vi "CODCr通讯.vi"() -> ()   [LabVIEW 2016, in "CODCr库.lvlib"]
uses:
  <vilib>/Plasmionique/MB Master/MB_Master/MB_Master.lvclass
  <vilib>/Plasmionique/MB Master/MB Master.lvlib
  <vilib>/Utility/config.llb/NI_LVConfig.lvlib
panel:
  out "状态告警区":u16[](array[numeric])
  out "测量数据区":u16[](array[numeric])
  in  "读取参数":bool
  in  "读取数据":bool
  in  "释放串口":bool
  in  "打开串口":bool
  out "队列中元素数量":i32
  out "元素":cluster{"命令":string}[](array[cluster])
  out "待处理插入数量":i32
  out "读取公式":u16[](array[numeric])
  out "读取参数":u16[](array[numeric])
  out "数据存储":u16[](array[numeric])
  out "通讯状态":bool
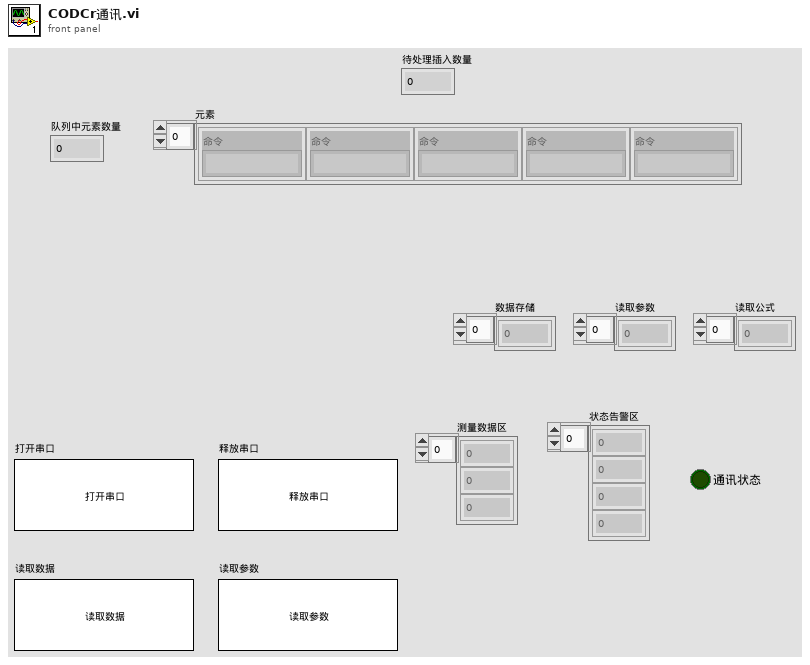
[diagram p1: front panel]
types:
  T1 = typedef "NI_LVConfig.lvlib/Config Data RefNum.ctl" = refnum<k1>
  T2 = cluster{"因子编码":u32, "单位":u16, "标样参考值":sgl, "水样数据时间":timestamp, "水样实测值":sgl, "水样数据标识":string, "标样数据时间":timestamp, "标样实测值":sgl, "标样数据标识":string, "空白数据时间":timestamp, "空白实测值":sgl, "空白数据标识":string, "零点核查数据时间":timestamp, "零点核查实测值":sgl, "零点核查数据标识":string, "跨度核查数据时间":timestamp, "跨度核查实测值":sgl, "跨度核查数据标识":string, "加标回收数据时间":timestamp, "加标回收实测值":sgl, "加标回收数据标识":string, "平行样数据时间":timestamp, "平行样实测值":sgl, "平行样数据标识":string}
  T3 = cluster{"系统时间":timestamp, "工作状态":enum16{"空闲", "水样测试", "标样核查", "零点核查", "跨度核查", "空白测试", "平行样测试", "加标回收", "空白校准", "标样校准", "初始化（清洗）"}, "测量模式":enum16{"待机", "连续模式", "周期模式", "定点模式", "受控模式", "手动模式"}, "告警代码":u16, "故障代码":u16, "日志代码":u16, "软件版本":u16, "F0":sgl, "F1":sgl, "F2":sgl, "F3":sgl, "T":sgl, "H":sgl, "id":u16, "flowid":u16, "量程":u16}
  T4 = cluster{"测量精度":u16, "消解温度":u16, "消解时长":u16, "量程下限":sgl, "量程上限":sgl, "曲线斜率K":sgl, "曲线斜率B":sgl, "标定日期":timestamp, "标液1浓度":sgl, "标液1测量过程值":sgl, "标液2浓度":sgl, "标液2测量过程值":sgl, "标液3浓度":sgl, "标液3测量过程值":sgl, "标液4浓度":sgl, "标液4测量过程值":sgl, "标液5浓度":sgl, "标液5测量过程值":sgl, "线性相关系数":sgl, "试剂余量":u32, "测量滴定值或吸光度":sgl, "空白校准时间":timestamp, "标样校准时间":timestamp, "检出限值":sgl, "校准系数":sgl, "设备系列号":string}
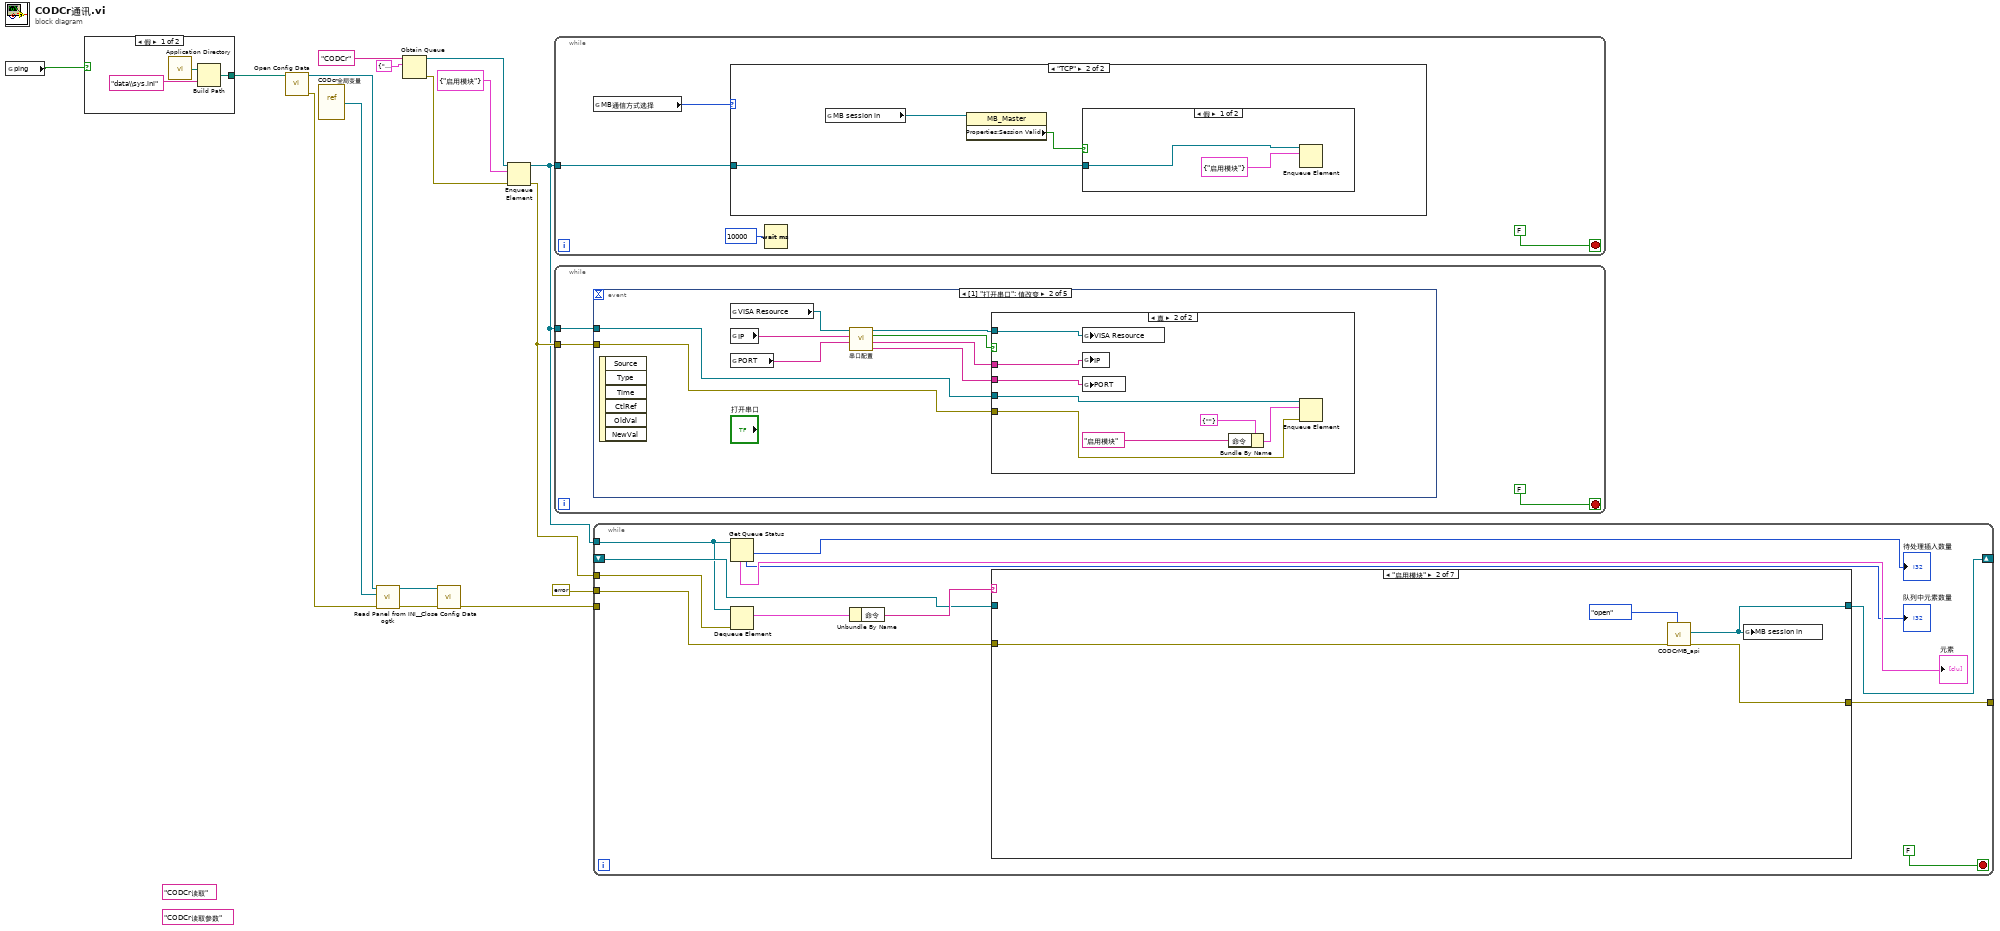
[diagram p0: block diagram]
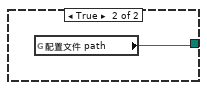
[diagram p2: hidden frame]
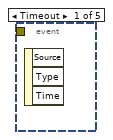
[diagram p5: hidden frame]
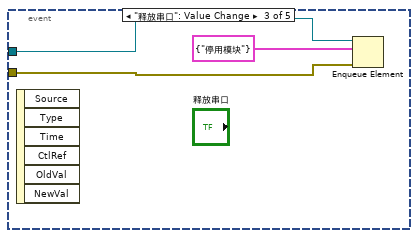
[diagram p7: hidden frame]
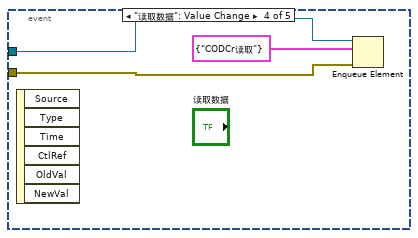
[diagram p8: hidden frame]
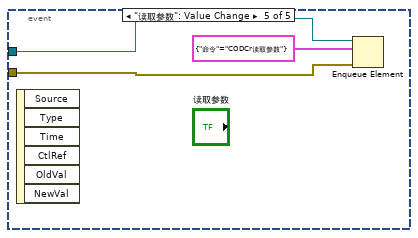
[diagram p9: hidden frame]
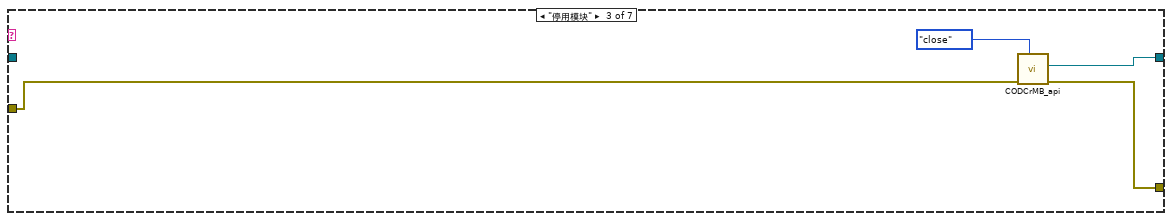
[diagram p11: hidden frame]
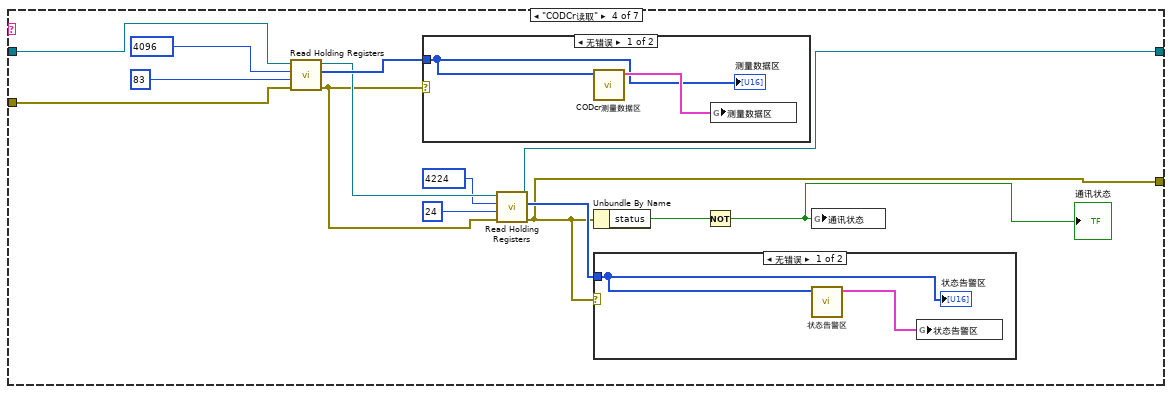
[diagram p12: hidden frame]
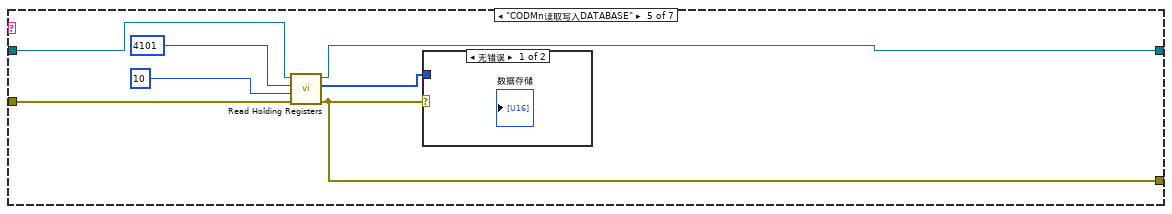
[diagram p15: hidden frame]
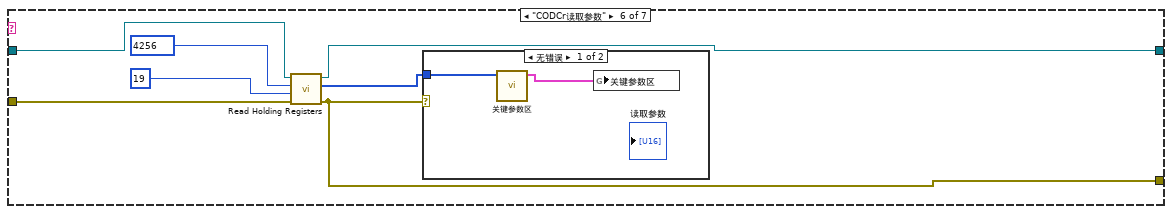
[diagram p17: hidden frame]
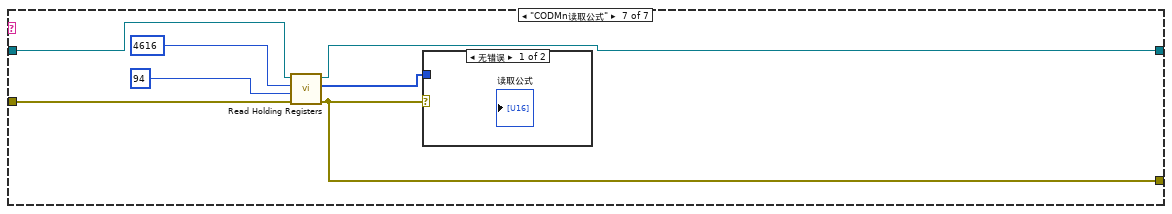
[diagram p19: hidden frame]
diagram:
  (unwired) "CODCr读取参数" ("名称（未命名）")
  (unwired) "CODCr读取" ("名称（未命名）")
  n1 = global read "CODcr全局变量.vi" "ping"() -> (w2:bool)
  n2 = case shown="假" w2 {
    tunnel: [w18 w20] -> w1
    frame False {
      n3 = call <vilib>:"Application Directory.vi"() -> ("Application Directory"=w19:path)
      n4 = Build Path(base path=w19, name or relative path="data\\sys.ini" ("名称或相对路径")) -> (appended path=w18:path)
    }
    frame True {
      n5 = global read "CODcr全局变量.vi" "配置文件 path"() -> (w20:path)
    }
  }
  n6 = call <vilib>:"Open Config Data.vi"("configuration file path"=w1) -> ("error out"=w7:errorcluster, "refnum"=w10:T1)  [unwired: 8 in, 1 out]
  n7 = vi-ref "CODcr全局变量.vi"() -> (w9:refnum<vi>)
  n8 = call <userlib>:"Read Panel from INI__ogtk.vi"("error in (no error)"=w7, "VI ref"=w9, "refnum"=w10) -> ("error out"=w6:errorcluster, "refnum out"=w8:T1)  [unwired: 7 in]
  n9 = Obtain Queue(name (unnamed)="CODCr" ("名称（未命名）"), element data type=cluster{"命令":string} {"命令"="启用模块"} ("元素")) -> (queue out=w13:refnum<queue>, error out=w12:errorcluster)  [unwired: 3 in, 1 out]
  n10 = call <vilib>:"Close Config Data.vi"("error in (no error)"=w6, "refnum"=w8) -> ("error out"=w3:errorcluster)  [unwired: 8 in, 1 out]
  n11 = Enqueue Element(queue=w13, element=cluster{"命令":string} {"命令"="启用模块"} ("元素"), error in (no error)=w12) -> (queue out=w4:refnum<queue>, error out=w5:errorcluster)  [unwired: 1 in, 1 out]
  n12 = while {
    tunnel: w4 -> [w24]
    stop <- FALSE stop-if-true
    n13 = global read "CODcr全局变量.vi" "MB通信方式选择"() -> (w22:enum16{"串口", "TCP"})
    n14 = case shown="\"TCP\"" w22 {
      tunnel: w24 -> [_ w25]
      frame "串口", Default {
      }
      frame "TCP" {
        n15 = global read "CODCr外部API.vi" "MB session in"() -> (w27:refnum<class "MB_Master.lvclass">)
        n16 = property class="MB_Master"(reference=w27) -> ("Properties:Session Valid"=w26:bool)  [unwired: 1 in, 2 out]
        n17 = case shown="假" w26 {
          tunnel: w25 -> [w29 _]
          frame False {
            n18 = Enqueue Element(queue=w29, element=cluster{"命令":string} {"命令"="启用模块"} ("元素")) -> ()  [unwired: 2 in, 3 out]
          }
          frame True {
          }
        }
      }
    }
    n19 = Wait (ms)(milliseconds to wait=u32 10000 ("等待时间（毫秒）")) -> ()  [unwired: 1 out]
  }
  n20 = while {
    tunnel: w4 -> [w31]
    tunnel: w5 -> [w30]
    stop <- FALSE stop-if-true
    n21 = event shown="[1] \"打开串口\": 值改变" {
      selector: _ -> [_ _ _ _ _]
      dyn-events: _ -> [_ _ _ _ _]
      timeout: _ -> [_ _ _ _ _]
      tunnel: w31 -> [_ w41 w52 w54 w57]
      tunnel: w30 -> [_ w40 w51 w53 w56]
      event Timeout {
        n22 = event-data() -> ()  [unwired: 1 in, 3 out]
      }
      event "打开串口": Value Change {
        n23 = event-data() -> ()  [unwired: 1 in, 6 out]
        n24 = global read "CODcr全局变量.vi" "VISA Resource"() -> (w39:refnum<visa-resource-name>)
        n25 = global read "CODcr全局变量.vi" "IP"() -> (w34:string)
        n26 = global read "CODcr全局变量.vi" "PORT"() -> (w33:string)
        n27 = call "串口配置.vi"("PORT"=w33, "IP"=w34, "请选择串口:"=w39) -> ("PORT 2"=w35:string, "IP 2"=w36:string, "确认 2"=w38:bool, "VISA资源名称 2"=w37:refnum<visa-resource-name>)  [unwired: 5 in]
        n28 = case shown="真" w38 {
          tunnel: w37 -> [_ w44]
          tunnel: w41 -> [_ w46]
          tunnel: w40 -> [_ w45]
          tunnel: w36 -> [_ w43]
          tunnel: w35 -> [_ w42]
          frame False {
          }
          frame True {
            n29 = global write "CODcr全局变量.vi" "VISA Resource"(w44) -> ()
            n30 = global write "CODcr全局变量.vi" "IP"(w43) -> ()
            n31 = global write "CODcr全局变量.vi" "PORT"(w42) -> ()
            n32 = Bundle By Name(cluster=cluster{"命令":string} {"命令"=""} ("元素"), "命令"="启用模块" ("名称（未命名）")) -> (w47:cluster{"命令":string})
            n33 = Enqueue Element(queue=w46, element=w47, error in (no error)=w45) -> ()  [unwired: 1 in, 3 out]
          }
        }
      }
      event "释放串口": Value Change {
        n34 = event-data() -> ()  [unwired: 1 in, 6 out]
        n35 = Enqueue Element(queue=w52, element=cluster{"命令":string} {"命令"="停用模块"} ("元素"), error in (no error)=w51) -> ()  [unwired: 1 in, 3 out]
      }
      event "读取数据": Value Change {
        n36 = event-data() -> ()  [unwired: 1 in, 6 out]
        n37 = Enqueue Element(queue=w54, element=cluster{"命令":string} {"命令"="CODCr读取"} ("元素"), error in (no error)=w53) -> ()  [unwired: 1 in, 3 out]
      }
      event "读取参数": Value Change {
        n38 = event-data() -> ()  [unwired: 1 in, 6 out]
        n39 = Enqueue Element(queue=w57, element=cluster{"命令":string} {"命令"="CODCr读取参数"} ("元素"), error in (no error)=w56) -> ()  [unwired: 1 in, 3 out]
      }
    }
  }
  n40 = while {
    tunnel: w4 -> [w62]
    tunnel: w5 -> [w69]
    tunnel: [w63] -> _
    shift-right: [w66] -> _
    shift-left: _ -> [w65]
    tunnel: errorcluster {"status"=FALSE, "code"=0, "source"=""} ("error out") -> [w64]
    tunnel: w3 -> [_]
    stop <- FALSE stop-if-true
    n41 = Get Queue Status(queue=w62) -> (# pending insert=→"待处理插入数量":i32, # elements in queue=→"队列中元素数量":i32, elements=→"元素":cluster{"命令":string}[])  [unwired: 2 in, 5 out]
    n42 = Dequeue Element(queue=w62, error in (no error)=w69) -> (element=w68:cluster{"命令":string})  [unwired: 1 in, 3 out]
    n43 = Unbundle By Name(w68) -> ("命令"=w67:string)
    n44 = case shown="\"启用模块\"" w67 {
      tunnel: [w72 w73 w77 w88 w101 w109 w118] -> w66
      tunnel: [w71 w76 w78 w81 w99 w108 w117] -> w63
      tunnel: w65 -> [w72 _ _ w94 w105 w112 w121]
      tunnel: w64 -> [w71 w74 w79 w93 w102 w111 w120]
      frame Default {
      }
      frame "启用模块" {
        n45 = call "CODCrMB_api.vi"("STEP"=enum16{"open", "read", "write", "close"}."open", "Error in"=w74) -> ("error out"=w76:errorcluster, "MB session out"=w73:refnum<class "MB_Master.lvclass">)  [unwired: 7 in, 1 out]
        n46 = global write "CODCr外部API.vi" "MB session in"(w73) -> ()
      }
      frame "停用模块" {
        n47 = call "CODCrMB_api.vi"("STEP"=enum16{"open", "read", "write", "close"}."close", "Error in"=w79) -> ("error out"=w78:errorcluster, "MB session out"=w77:refnum<class "MB_Master.lvclass">)  [unwired: 7 in, 1 out]
      }
      frame "CODCr读取" {
        n48 = call <vilib>:"Read Holding Registers.vi"("error in (no error)"=w93, "quantity"=u16 83 ("number of holding registers"), "starting address"=u16 4096, "MB session in"=w94) -> ("error out"=w90:errorcluster, "Registers"=w92:u16[], "MB session out"=w91:refnum<class "MB_Master.lvclass">)  [unwired: 5 in]
        n49 = case shown="无错误" w90 {
          tunnel: w92 -> [w97 _]
          frame No Error {
            n50 = call "CODcr测量数据区.vi"("数组"=w97) -> ("测量数据区"=w98:T2)  [unwired: 10 in]
            n51 = global write "CODcr全局变量.vi" "测量数据区"(w98) -> ()
            "测量数据区" <- w97
          }
          frame Error {
          }
        }
        n52 = call <vilib>:"Read Holding Registers.vi"("error in (no error)"=w90, "quantity"=u16 24 ("number of holding registers"), "starting address"=u16 4224, "MB session in"=w91) -> ("error out"=w81:errorcluster, "Registers"=w89:u16[], "MB session out"=w88:refnum<class "MB_Master.lvclass">)  [unwired: 5 in]
        n53 = Unbundle By Name(w81) -> ("status"=w82:bool)
        n54 = case shown="无错误" w81 {
          tunnel: w89 -> [w95 _]
          frame No Error {
            n55 = call "状态告警区.vi"("数组"=w95) -> ("状态告警区"=w96:T3)  [unwired: 10 in]
            n56 = global write "CODcr全局变量.vi" "状态告警区"(w96) -> ()
            "状态告警区" <- w95
          }
          frame Error {
          }
        }
        n57 = Not(x=w82) -> (.not. x?=w83:bool)
        "通讯状态" <- w83
        n58 = global write "CODcr全局变量.vi" "通讯状态"(w83) -> ()
      }
      frame "CODMn读取写入DATABASE" {
        n59 = call <vilib>:"Read Holding Registers.vi"("error in (no error)"=w102, "quantity"=u16 10 ("number of holding registers"), "starting address"=u16 4101, "MB session in"=w105) -> ("error out"=w99:errorcluster, "Registers"=w100:u16[], "MB session out"=w101:refnum<class "MB_Master.lvclass">)  [unwired: 5 in]
        n60 = case shown="无错误" w99 {
          tunnel: w100 -> [_ _]
          frame No Error {
          }
          frame Error {
          }
        }
      }
      frame "CODCr读取参数" {
        n61 = call <vilib>:"Read Holding Registers.vi"("error in (no error)"=w111, "quantity"=u16 19 ("number of holding registers"), "starting address"=u16 4256, "MB session in"=w112) -> ("error out"=w108:errorcluster, "Registers"=w110:u16[], "MB session out"=w109:refnum<class "MB_Master.lvclass">)  [unwired: 5 in]
        n62 = case shown="无错误" w108 {
          tunnel: w110 -> [w113 _]
          frame No Error {
            n63 = call "关键参数区.vi"("数组"=w113) -> ("关键参数区"=w114:T4)  [unwired: 10 in]
            n64 = global write "CODcr全局变量.vi" "关键参数区"(w114) -> ()
          }
          frame Error {
          }
        }
      }
      frame "CODMn读取公式" {
        n65 = call <vilib>:"Read Holding Registers.vi"("error in (no error)"=w120, "quantity"=u16 94 ("number of holding registers"), "starting address"=u16 4616, "MB session in"=w121) -> ("error out"=w117:errorcluster, "Registers"=w119:u16[], "MB session out"=w118:refnum<class "MB_Master.lvclass">)  [unwired: 5 in]
        n66 = case shown="无错误" w117 {
          tunnel: w119 -> [_ _]
          frame No Error {
          }
          frame Error {
          }
        }
      }
    }
  }
